vi "onHttpPost (Multipart).vi"(8 "error in":errorcluster, 10 "httpRequest":refnum<class "httpRequest.lvclass">, 11 "advanced-http-client in":refnum<class "advanced-http-client.lvclass">) -> (0 "error out":errorcluster, 2 "httpResponse":refnum<class "httpResponse.lvclass">, 3 "advanced-http-client out":refnum<class "advanced-http-client.lvclass">)   [LabVIEW 2020, in "HttpClient.NiAdvanced.lvlib" / "advanced-http-client.lvclass"]
uses:
  advanced-http-client.lvclass
  advanced-http-client.lvclass/advanced-http-client.ctl
  <vilib>/NI/Advanced HTTP Client/Session.lvclass
  http-client-pkg/httpRequest/httpRequest.lvclass
  <vilib>/NI/Advanced HTTP Client/POST (Multipart).vi
  http-client-pkg/httpResponse/httpResponse.lvclass
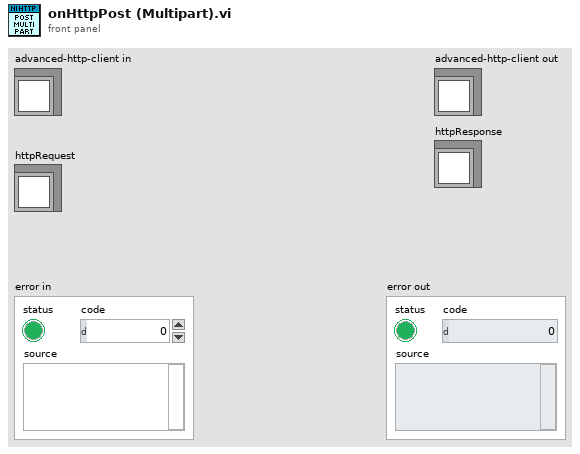
[diagram p1: front panel]
types:
  T1 = typedef "httpClient.lvlib/httpRequest.lvclass/Multipart data -- cluster.ctl" = cluster{"Name":string, "Value":string, "File":path, "Filename":string, "MIME type":string}
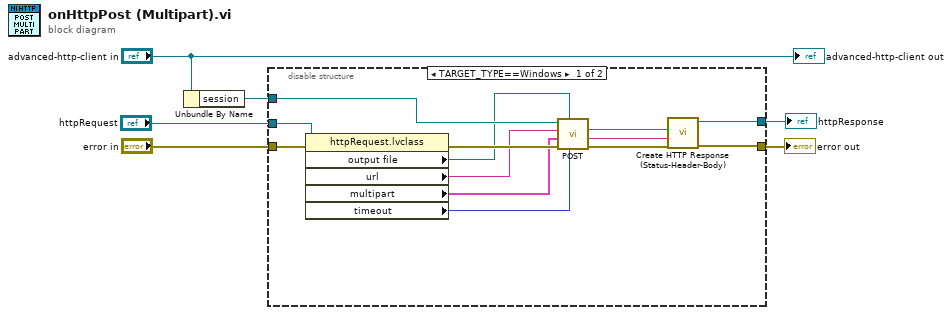
[diagram p0: block diagram]
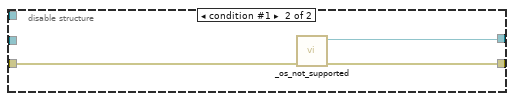
[diagram p2: hidden frame]
diagram:
  n1 = Unbundle By Name("advanced-http-client in") -> ("session"=w5:refnum<class "Session.lvclass">)
  n2 = disable-structure shown="TARGET_TYPE==Windows" {
    disable-tunnel: w5 -> [w19 _]
    disable-tunnel: "error in" -> [w17 w22]
    disable-tunnel: [w10 w21] -> w3
    disable-tunnel: [w9 w20] -> w2
    disable-tunnel: "httpRequest" -> [w16 _]
    frame condition #0 (active) {
      n3 = property class="httpRequest.lvclass"(reference=w16, error in=w17) -> (error out=w18:errorcluster, "output file"=w15:path, "url"=w14:string, "multipart"=w12:T1[], "timeout"=w13:i32)  [unwired: 1 out]
      n4 = call-poly <vilib>:"POST.vi"("timeout"=w13, "output file"=w15, "error in"=w18, "data"=w12, "url"=w14, "session in"=w19) -> ("error out"=w11:errorcluster, "body"=w7:string, "headers"=w8:string)  [unwired: 1 in, 2 out]
      n5 = call "Create HTTP Response (Status-Header-Body).vi"("error in"=w11, "body"=w7, "Headers w/ status line(s)"=w8) -> ("error out"=w10:errorcluster, "httpResponse out"=w9:refnum<class "httpResponse.lvclass">)  [unwired: 7 in]
    }
    frame condition #1 {
      n6 = call "_os_not_supported.vi"("error in (no error)"=w22) -> ("error out"=w21:errorcluster, "httpResponse"=w20:refnum<class "httpResponse.lvclass">)  [unwired: 9 in]
    }
  }
  "error out" <- w3
  "httpResponse" <- w2
  "advanced-http-client out" <- "advanced-http-client in"
